vi "Reward.vi"() -> (3 "reward":dbl=0.892455449826875)   [LabVIEW 2017]
uses:
  <vilib>/Analysis/_algsub.llb/Real Vector Norm.vi
  <vilib>/Analysis/NI_AALPro.lvlib
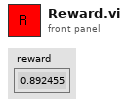
[diagram p1: front panel]
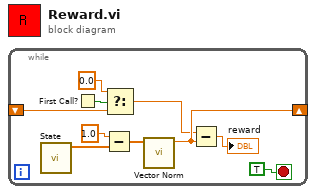
[diagram p0: block diagram]
diagram:
  n1 = while {
    shift-right: [w5] -> _
    shift-left: _ -> [w4]
    stop <- TRUE stop-if-true
    n2 = call "State.vi"() -> ("state"=w8:dbl[])  [unwired: 11 in]
    n3 = First Call?() -> (First Call?: T/F=w9:bool)
    n4 = Subtract(x=1.0, y=w8) -> (x-y=w6:dbl[])
    n5 = Select(t=0.0, s=w9, f=w4) -> (s? t:f=w2:dbl)
    n6 = call-poly <vilib>:"Vector Norm.vi"("Input Vector"=w6) -> ("norm"=w5:dbl)  [unwired: 9 in, 1 out]
    n7 = Subtract(x=w2, y=w5) -> (x-y=→"reward":dbl)
  }
